vi "Read position, mm.vi"(8 "error in (no error)":errorcluster, 10 "axis":i16, 11 "DelayLineSimulation in":refnum<class "DLEmulate.lvclass">) -> (0 "error out":errorcluster, 2 "position, mm":dbl, 3 "DelayLineSimulation out":refnum<class "DLEmulate.lvclass">)   [LabVIEW 2018, in "DLEmulate.lvclass"]
uses:
  DLEmulate.lvclass
  DLEmulate.lvclass/DLEmulate.ctl
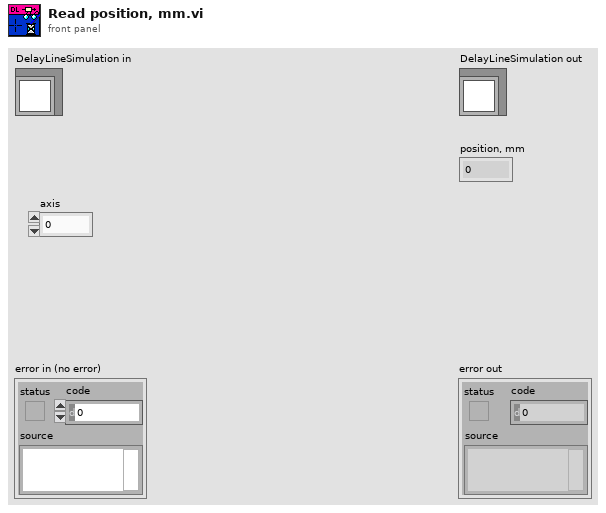
[diagram p1: front panel]
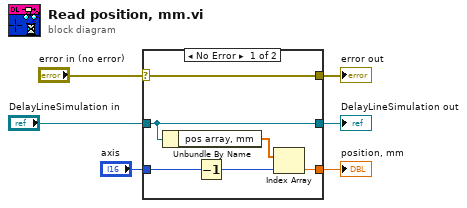
[diagram p0: block diagram]
diagram:
  n1 = case shown="No Error" "error in (no error)" {
    selector: "error in (no error)" -> [w12 w13]
    tunnel: [w12 w13] -> w5
    tunnel: [w11 w14] -> w3
    tunnel: "DelayLineSimulation in" -> [w11 w14]
    tunnel: [w8 _] -> w2
    tunnel: "axis" -> [w9 _]
    frame No Error {
      n2 = Unbundle By Name(w11) -> ("pos array, mm"=w10:dbl[])
      n3 = Decrement(x=w9) -> (x-1=w7:i16)
      n4 = Index Array(array=w10, index=w7) -> (element=w8:dbl)
    }
    frame Error {
    }
  }
  "error out" <- w5
  "DelayLineSimulation out" <- w3
  "position, mm" <- w2
